vi "Calculate Fall Time.vi"(7 "Waveform Array":waveform(dbl)[](array[waveform]), 9 "Digitizer Channel (1-4)":i32) -> (8 "Fall Time":dbl)   [LabVIEW 2010]
uses:
  <vilib>/measure/mamon.llb/Trigger Detection for 1 Channel.vi
  <vilib>/measure/NI_MAPro.lvlib
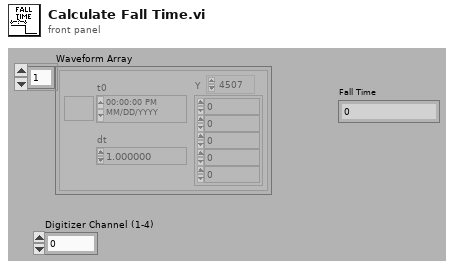
[diagram p1: front panel]
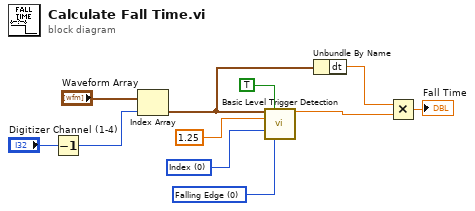
[diagram p0: block diagram]
diagram:
  w6 = u16 0 items=["Falling Edge", "Rising Edge"] ("trigger slope")
  w7 = u16 0 items=["Index", "Time"] ("location mode")
  n1 = Decrement(x="Digitizer Channel (1-4)") -> (x-1=w9:i32)
  n2 = Index Array(array="Waveform Array", index=w9) -> (element=w4:waveform(dbl))
  n3 = call-poly <vilib>:"Basic Level Trigger Detection.vi"("signal in"=w4, "reset"=TRUE, "level"=1.25, "location mode"=w7, "trigger slope"=w6) -> ("trigger location"=w2:dbl)  [unwired: 8 in, 2 out]
  n4 = Unbundle By Name(w4) -> ("dt"=w1:dbl)
  n5 = Multiply(x=w1, y=w2) -> (x*y=→"Fall Time":dbl)
